vi "BNC555.evt call Chan Gating On or Off.vi"(0 "i ref in":refnum<vi>, 2 "Generator Instance":string="N/A", 3 "Channel":i32(ring)=1 items=["System (To)", "Channel A", "Channel B", "Channel C", "Channel D", "Channel E", "Channel F", "Channel G", "Channel H"], 4 "Gating State":bool, 5 "error in (no error)":errorcluster) -> (14 "i ref out":refnum<vi>, 19 "error out":errorcluster)   [LabVIEW 2014, in "BNC555.lvlib"]
doc: "This VI sends a simple event call to the wired BNC555."
uses:
  BNC555.lvlib
  CSCore/CSSystem/CoreLib/CoreLib.short 2 byte array.vi
  CSCore/CSSystem/CoreLib/CoreLib.int 2 byte array.vi
  CSCore/CSSystem/CoreLib/CoreLib.lvlib
  CSCore/BaseProcess/BaseProcess.lvlib
panel:
  # "On\nOff"
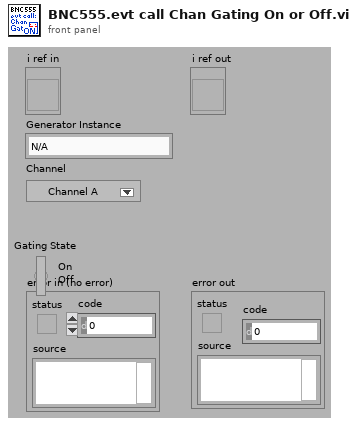
[diagram p1: front panel]
types:
  T1 = typedef "CoreDefs.rawDataType.ctl" = i8[]
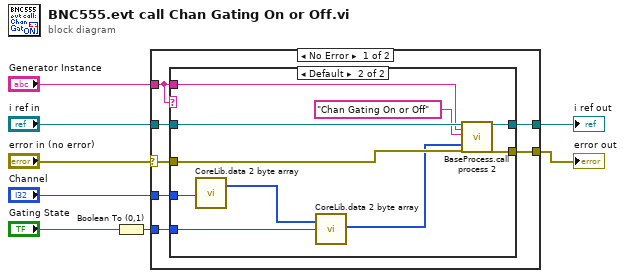
[diagram p0: block diagram]
diagram:
  n1 = Boolean To (0,1)(Boolean="Gating State") -> (0, 1=w3:i16)
  n2 = case shown="No Error" "error in (no error)" {
    selector: "error in (no error)" -> [w12 w28]
    tunnel: [w15 w29] -> w7
    tunnel: [w14 w28] -> w6
    tunnel: "i ref in" -> [w13 w29]
    tunnel: "Generator Instance" -> [w11 _]
    tunnel: "Channel" -> [w10 _]
    tunnel: w3 -> [w9 _]
    frame No Error {
      n3 = case shown="Default" w11 {
        tunnel: [w17 w27] -> w15
        tunnel: [w16 w26] -> w14
        tunnel: w13 -> [w17 w25]
        tunnel: w11 -> [_ w24]
        tunnel: w12 -> [w16 w22]
        tunnel: w10 -> [_ w21]
        tunnel: w9 -> [_ w20]
        frame "N/A" {
        }
        frame Default {
          n4 = call-poly "CoreLib.data 2 byte array.vi"("i32"=w21) -> ("byteArray out"=w19:T1)  [unwired: 18 in]
          n5 = call-poly "CoreLib.data 2 byte array.vi"("byteArray"=w19, "i16"=w20) -> ("byteArray out"=w18:T1)  [unwired: 17 in]
          n6 = call "BaseProcess.call process 2.vi"("i ref in"=w25, "Object"=w24, "Selector"="Chan Gating On or Off", "Data"=w18, "error in (no error)"=w22) -> ("i ref out"=w27:refnum<vi>, "error out"=w26:errorcluster)  [unwired: 13 in]
        }
      }
    }
    frame Error {
    }
  }
  "error out" <- w6
  "i ref out" <- w7
